vi "Size Calculator.vi"(11 "Bytes":u64) -> (1 "Gigabytes":dbl, 2 "Megabytes":dbl, 3 "Kilobytes":dbl)   [LabVIEW 2014, in "TDMS Logger.lvlib" / "TDMS Logger.lvclass"]
uses:
  TDMS Logger.lvclass
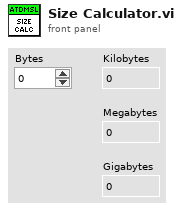
[diagram p1: front panel]
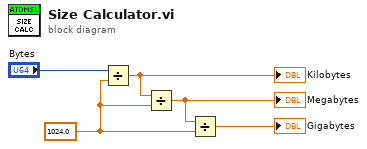
[diagram p0: block diagram]
diagram:
  w3 = 1024.0 ("y")
  n1 = Divide(x="Bytes", y=w3) -> (x/y=w2:dbl)
  "Kilobytes" <- w2
  n2 = Divide(x=w2, y=w3) -> (x/y=w4:dbl)
  "Megabytes" <- w4
  n3 = Divide(x=w4, y=w3) -> (x/y=→"Gigabytes":dbl)
